vi "openDocuement.vi"(8 "error in (no error)":errorcluster, 11 "MS-Excel in":refnum<class "MS-Excel.lvclass">) -> (0 "error out":errorcluster, 3 "MS-Excel out":refnum<class "MS-Excel.lvclass">)   [LabVIEW 2020, in "LabVIEW NPOI.lvlib" / "MS-Excel.lvclass"]
doc: "Create a new Excel workbook at the FilePath location. If the location already contains an excel workbook with the same name then that file is overwritten without warning.\n\nThe workbook will contain 1 sheet named 'Sheet1'. The first row is selected."
uses:
  MS-Excel.lvclass
  D:/Benjamin/Documents/Perso/Code/WC/LabVIEW_NPOI/src/LabVIEW NPOI/Document/Document.lvclass
  Document/Document.lvclass/Document.ctl
  D:/Benjamin/Documents/Perso/Code/WC/LabVIEW_NPOI/lib/NPOI 2.1.1/NPOI.OOXML.dll
  lib/NPOI 2.1.1/NPOI.OOXML.dll
  MS-Excel.lvclass/MS-Excel.ctl
  Document/Get FilePath.vi
  Document/Document.lvclass
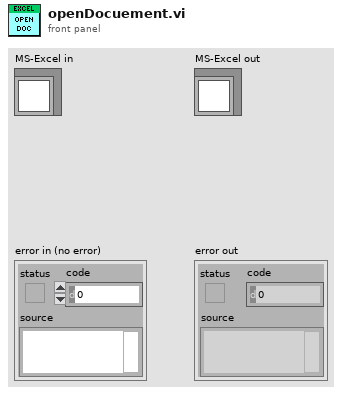
[diagram p1: front panel]
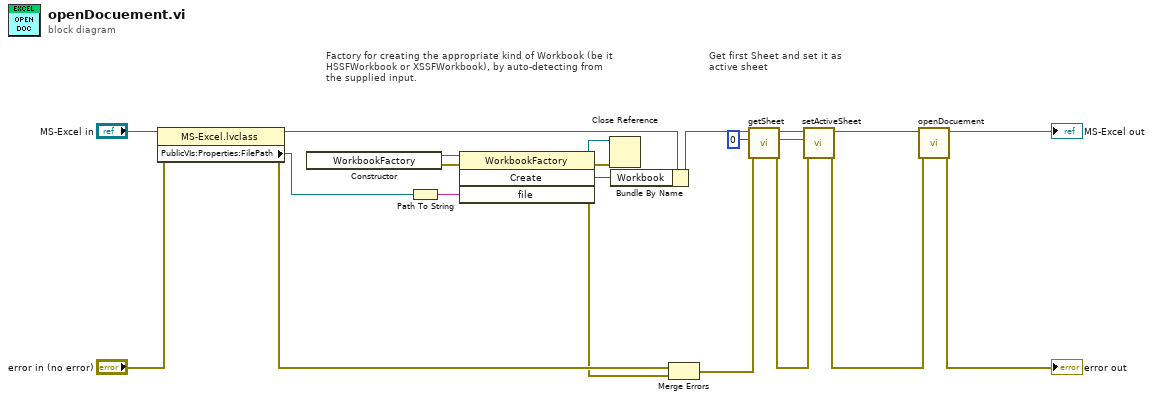
[diagram p0: block diagram]
diagram:
  # "Get first Sheet and set it as\nactive sheet"
  # "Factory for creating the appropriate kind of Workbook (be it HSSFWorkbook or XSSFWorkbook), by auto-detecting from the supplied input."
  n1 = property class="MS-Excel.lvclass"(reference="MS-Excel in", error in="error in (no error)") -> (reference out=w14:refnum<class "MS-Excel.lvclass">, error out=w13:errorcluster, "PublicVIs:Properties:FilePath"=w11:path)
  n2 = constructor class="WorkbookFactory"() -> (reference out=w21:refnum<k24>, error out=w20:errorcluster)  [unwired: 3 in, 1 out]
  n3 = Path To String(path=w11) -> (string=w10:string)
  n4 = invoke class="WorkbookFactory" method="Create"(reference=w21, error in=w20, "file"=w10) -> (reference out=w19:refnum<k24>, error out=w12:errorcluster, "Create"=w18:refnum<k24>)  [unwired: 1 in, 1 out]
  n5 = Close Reference(reference=w19, error in (no error)=w12) -> ()  [unwired: 1 out]
  n6 = Bundle By Name(cluster=w14, "Workbook"=w18) -> (w17:refnum<class "MS-Excel.lvclass">)
  n7 = Merge Errors(w13, w12) -> (w16:errorcluster)
  n8 = call-dynamic "getSheet.vi"("error in (no error)"=w16, "Sheet Index"=0, "MS-Excel in"=w17) -> ("error out"=w7:errorcluster, "Sheet Ref"=w8:refnum<k24>, "MS-Excel out"=w9:refnum<class "MS-Excel.lvclass">)  [unwired: 6 in]
  n9 = call-dynamic "setActiveSheet.vi"("error in (no error)"=w7, "Sheet Ref"=w8, "MS-Excel in"=w9) -> ("error out"=w2:errorcluster, "MS-Excel out"=w4:refnum<class "MS-Excel.lvclass">)  [unwired: 7 in]
  n10 = call-parent "openDocuement.vi"("error in (no error)"=w2, "Document in"=w4) -> ("error out"=→"error out":errorcluster, "Document out"=→"MS-Excel out":refnum<class "MS-Excel.lvclass">)  [unwired: 8 in]
